vi "Periodic Tasks.vi"(8 "error in":errorcluster) -> ()   [LabVIEW 2013]
doc: "This VI runs in parallel to other tasks. It can contain as many user-defined periodic loops as you need. These can carry out PID or other sorts of timed response."
uses:
  Systems/Compressor/Compressor.lvclass
  <vilib>/Rock Robotics/SystemInterfaces/Utilities/FPGA_UtilitiesLED Source.ctl
  <vilib>/Rock Robotics/SystemInterfaces/Utilities/FPGA_UtilitiesLED State.ctl
  Systems/Blocker/Blocker.lvclass
  Commands/Command/Command.lvclass
  Systems/Catapult/Catapult.lvclass
  Systems/GrabberArms/GrabberArms.lvclass
  Systems/GrabberWheels/GrabberWheels.lvclass
  Systems/Shifter/Shifter.lvclass
  Systems/DriveMotors/DriveMotors.lvclass
  Robot Global Data.vi
panel:
  in  "Blocker Wait":u32=250
  in  "Catapult Wait":u32=75
  in  "Grabber Wait":u32=150
  in  "DriveMotors Wait":u32=75
  out "Blocker Enabled":bool
  out "Shifter Enabled":bool
  out "DML Enabled":bool
  out "DMR Enabled":bool
  out "Grabber Arms Enabled":bool
  out "Grabber Wheels Enabled":bool
  out "Catapult Enabled?":bool
  in  "System Info":T1(tab)
  out "DML":string
  out "DMR":string
  out "DML Distance":dbl
  out "DML Rate":dbl
  out "DMR Rate":dbl
  out "DMR Distance":dbl
  out "Shifter":string
  out "CT":string
  out "Catapult Switch Real Value":bool
  out "GA Switch Real Value":bool
  out "GA":string
  out "GW":string
  out "Blocker":string
  in  "Enable Catapult":bool=TRUE
  in  "Enable Grabber Wheels":bool=TRUE
  in  "Enable Grabber Arms":bool=TRUE
  in  "Enable Shifter":bool=TRUE
  in  "Enable DMR":bool=TRUE
  in  "Enable DML":bool=TRUE
  in  "Semaphore Timeout":i32=-1
  # "Manual Enables(Currently Disabled)"
  # "Dashboard Enables"
  # "Value which comes out of the DIO, which is inverted in the code"
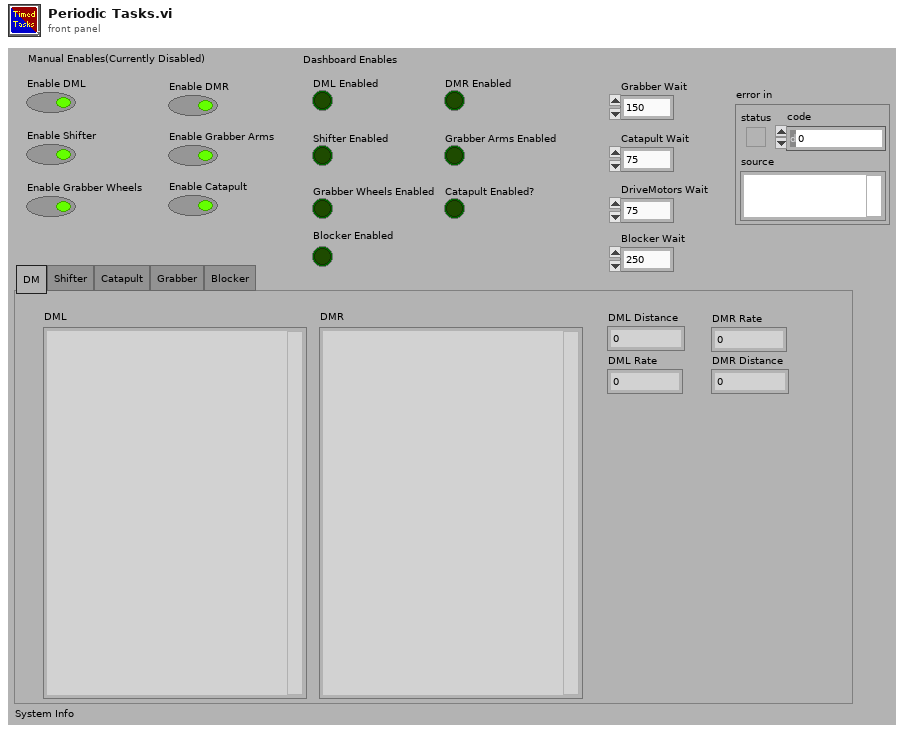
[diagram p1: front panel]
types:
  T1 = enum32{"DM", "Shifter", "Catapult", "Grabber", "Blocker"}
  T2 = typedef "Semaphore RefNum" = refnum<k1>
  T3 = typedef "WPI_DigitalInputDevRef.ctl" = cluster{"DevStatus":errorcluster, "DIO Channel":T4, "Digital Module":T5}
  T4 = typedef "FPGA_DIOChannel.ctl" = enum8{"DIO 1", "DIO 2", "DIO 3", "DIO 4", "DIO 5", "DIO 6", "DIO 7", "DIO 8", "DIO 9", "DIO 10", "DIO 11", "DIO 12", "DIO 13", "DIO 14", "Invalid"}
  T5 = typedef "FPGA_TypedefDigitalModule.ctl" = enum16{"Digital Module 1", "Digital Module 2"}
  T6 = typedef "FPGA_UtilitiesLED State.ctl" = enum16{"Off", "On", "Toggle"}
  T7 = typedef "FPGA_UtilitiesLED Source.ctl" = enum16{"User LED", "FPGA LED"}
  T8 = typedef "WPI_CompressorDevRef.ctl" = cluster{"DevStatus":errorcluster, "DigitalInputDevRef":T3, "RelayDevRef":T9}
  T9 = typedef "WPI_RelayDevRef.ctl" = cluster{"DevStatus":errorcluster, "Relay Channel":T10, "Digital Module":T5, "Relay Direction":T11}
  T10 = typedef "FPGA_DIORelayChannel.ctl" = enum8{"Relay 1", "Relay 2", "Relay 3", "Relay 4", "Relay 5", "Relay 6", "Relay 7", "Relay 8", "Invalid"}
  T11 = typedef "WPI_RelayDirection.ctl" = enum16{"Both directions", "Forward only", "Reverse only"}
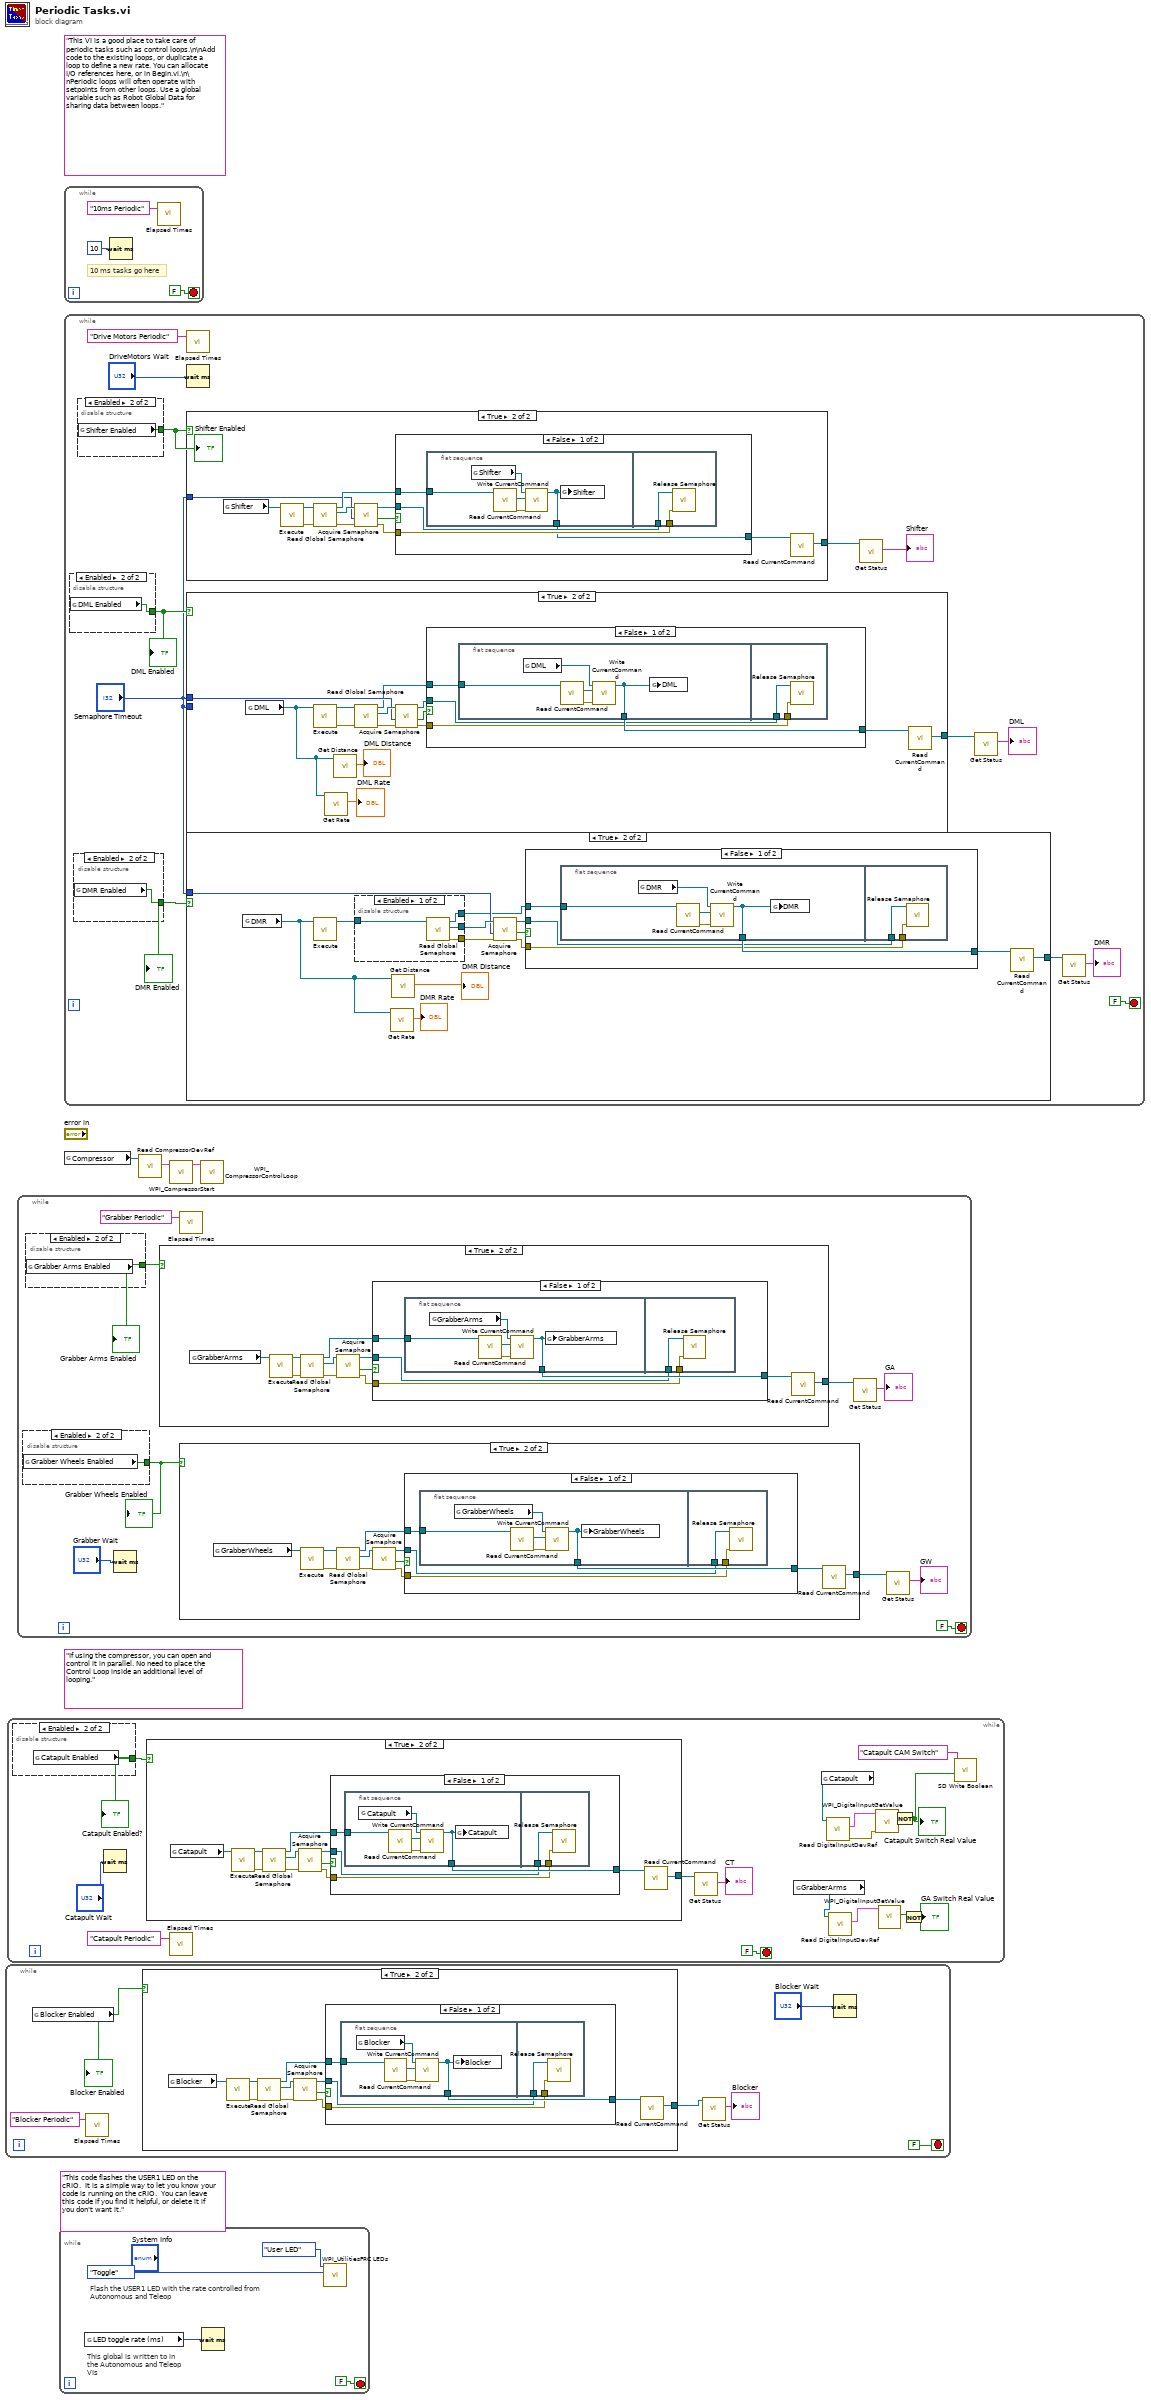
[diagram p0: block diagram]
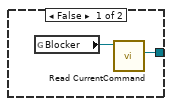
[diagram p2: hidden frame]
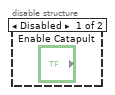
[diagram p4: hidden frame]
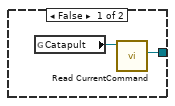
[diagram p5: hidden frame]
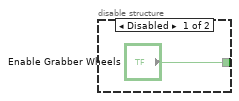
[diagram p7: hidden frame]
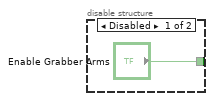
[diagram p8: hidden frame]
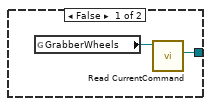
[diagram p9: hidden frame]
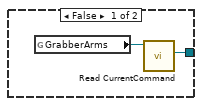
[diagram p11: hidden frame]
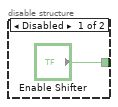
[diagram p13: hidden frame]
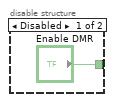
[diagram p14: hidden frame]
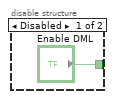
[diagram p15: hidden frame]
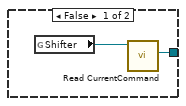
[diagram p16: hidden frame]
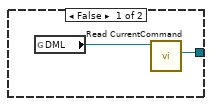
[diagram p18: hidden frame]
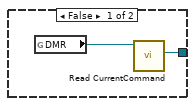
[diagram p20: hidden frame]
diagram:
  (unwired) "If using the compressor, you can open and control it in parallel. No need to place the Control Loop inside an additional level of looping."
  (unwired) "This code flashes the USER1 LED on the cRIO.  It is a simple way to let you know your code is running on the cRIO.  You can leave this code if you find it helpful, or delete it if you don't want it."
  (unwired) "This VI is a good place to take care of periodic tasks such as control loops.\n\nAdd code to the existing loops, or duplicate a loop to define a new rate. You can allocate I/O references here, or in Begin.vi.\n\nPeriodic loops will often operate with setpoints from other loops. Use a global variable such as Robot Global Data for sharing data between loops."
  n1 = while {
    stop <- FALSE stop-if-true
    n2 = global read "Robot Global Data.vi" "Blocker Enabled"() -> (w8:bool)
    "Blocker Enabled" <- w8
    n3 = call "Elapsed Times.vi"("Call Name"="Blocker Periodic") -> ()  [unwired: 2 in, 1 out]
    n4 = case shown="True" w8 {
      tunnel: [w10 w13] -> w7
      frame False {
        n5 = global read "Robot Global Data.vi" "Blocker"() -> (w11:refnum<class "Blocker.lvclass">)
        n6 = call-dynamic "Read CurrentCommand.vi"("System in"=w11) -> ("Command.lvclass"=w10:refnum<class "Command.lvclass">)  [unwired: 8 in, 2 out]
      }
      frame True {
        n7 = global read "Robot Global Data.vi" "Blocker"() -> (w22:refnum<class "Blocker.lvclass">)
        n8 = call-dynamic "Execute.vi"("System in"=w22) -> ("error out"=w20:errorcluster, "System out"=w21:refnum<class "Blocker.lvclass">)  [unwired: 9 in]
        n9 = call-dynamic "Read Global Semaphore.vi"("error in (no error)"=w20, "System in"=w21) -> ("error out"=w18:errorcluster, "semaphore"=w19:T2, "System out"=w16:refnum<class "Blocker.lvclass">)  [unwired: 7 in]
        n10 = call <vilib>:"Acquire Semaphore.vi"("error in (no error)"=w18, "semaphore"=w19) -> ("error out"=w15:errorcluster, "timed out"=w17:bool, "semaphore out"=w14:T2)  [unwired: 3 in]
        n11 = case shown="False" w17 {
          tunnel: w16 -> [w26 w34]
          tunnel: w15 -> [w23 _]
          tunnel: w14 -> [w24 _]
          tunnel: [w25 w34] -> w12
          frame False {
            n12 = flat-sequence {
              tunnel: w26 -> [w31]
              tunnel: [w27] -> w25
              tunnel: w24 -> [w33]
              tunnel: w23 -> [w32]
              frame #0 {
                n13 = global read "Robot Global Data.vi" "Blocker"() -> (w29:refnum<class "Blocker.lvclass">)
                n14 = call-dynamic "Read CurrentCommand.vi"("System in"=w31) -> ("error out"=w28:errorcluster, "Command.lvclass"=w30:refnum<class "Command.lvclass">)  [unwired: 8 in, 1 out]
                n15 = call-dynamic "Write CurrentCommand.vi"("error in (no error)"=w28, "Command.lvclass"=w30, "System in"=w29) -> ("System out"=w27:refnum<class "Blocker.lvclass">)  [unwired: 7 in, 1 out]
                n16 = global write "Robot Global Data.vi" "Blocker"(w27) -> ()
              }
              frame #1 {
                n17 = call <vilib>:"Release Semaphore.vi"("error in (no error)"=w32, "semaphore"=w33) -> ()  [unwired: 4 in, 2 out]
              }
            }
          }
          frame True {
          }
        }
        n18 = call-dynamic "Read CurrentCommand.vi"("System in"=w12) -> ("Command.lvclass"=w13:refnum<class "Command.lvclass">)  [unwired: 8 in, 2 out]
      }
    }
    n19 = call-dynamic "Get Status.vi"("Command in"=w7) -> ("Status"=→"Blocker":string)  [unwired: 8 in, 2 out]
    n20 = Wait (ms)(milliseconds to wait="Blocker Wait") -> ()  [unwired: 1 out]
  }
  n21 = while {
    stop <- FALSE stop-if-true
    n22 = disable-structure shown="Enabled" {
      disable-tunnel: [_ w51] -> w37
      frame Disabled {
      }
      frame Enabled {
        n23 = global read "Robot Global Data.vi" "Catapult Enabled"() -> (w51:bool)
      }
    }
    "Catapult Enabled?" <- w37
    n24 = Wait (ms)(milliseconds to wait="Catapult Wait") -> ()  [unwired: 1 out]
    n25 = case shown="True" w37 {
      tunnel: [w52 w55] -> w46
      frame False {
        n26 = global read "Robot Global Data.vi" "Catapult"() -> (w53:refnum<class "Catapult.lvclass">)
        n27 = call-dynamic "Read CurrentCommand.vi"("System in"=w53) -> ("Command.lvclass"=w52:refnum<class "Command.lvclass">)  [unwired: 8 in, 2 out]
      }
      frame True {
        n28 = global read "Robot Global Data.vi" "Catapult"() -> (w64:refnum<class "Catapult.lvclass">)
        n29 = call-dynamic "Execute.vi"("System in"=w64) -> ("error out"=w62:errorcluster, "System out"=w63:refnum<class "Catapult.lvclass">)  [unwired: 9 in]
        n30 = call-dynamic "Read Global Semaphore.vi"("error in (no error)"=w62, "System in"=w63) -> ("error out"=w60:errorcluster, "semaphore"=w61:T2, "System out"=w58:refnum<class "Catapult.lvclass">)  [unwired: 7 in]
        n31 = call <vilib>:"Acquire Semaphore.vi"("error in (no error)"=w60, "semaphore"=w61) -> ("error out"=w57:errorcluster, "timed out"=w59:bool, "semaphore out"=w56:T2)  [unwired: 3 in]
        n32 = case shown="False" w59 {
          tunnel: w58 -> [w68 w76]
          tunnel: w57 -> [w65 _]
          tunnel: w56 -> [w66 _]
          tunnel: [w67 w76] -> w54
          frame False {
            n33 = flat-sequence {
              tunnel: w68 -> [w73]
              tunnel: [w69] -> w67
              tunnel: w66 -> [w75]
              tunnel: w65 -> [w74]
              frame #0 {
                n34 = global read "Robot Global Data.vi" "Catapult"() -> (w71:refnum<class "Catapult.lvclass">)
                n35 = call-dynamic "Read CurrentCommand.vi"("System in"=w73) -> ("error out"=w70:errorcluster, "Command.lvclass"=w72:refnum<class "Command.lvclass">)  [unwired: 8 in, 1 out]
                n36 = call-dynamic "Write CurrentCommand.vi"("error in (no error)"=w70, "Command.lvclass"=w72, "System in"=w71) -> ("System out"=w69:refnum<class "Catapult.lvclass">)  [unwired: 7 in, 1 out]
                n37 = global write "Robot Global Data.vi" "Catapult"(w69) -> ()
              }
              frame #1 {
                n38 = call <vilib>:"Release Semaphore.vi"("error in (no error)"=w74, "semaphore"=w75) -> ()  [unwired: 4 in, 2 out]
              }
            }
          }
          frame True {
          }
        }
        n39 = call-dynamic "Read CurrentCommand.vi"("System in"=w54) -> ("Command.lvclass"=w55:refnum<class "Command.lvclass">)  [unwired: 8 in, 2 out]
      }
    }
    n40 = call "Elapsed Times.vi"("Call Name"="Catapult Periodic") -> ()  [unwired: 2 in, 1 out]
    n41 = call-dynamic "Get Status.vi"("Command in"=w46) -> ("Status"=→"CT":string)  [unwired: 8 in, 2 out]
    n42 = global read "Robot Global Data.vi" "GrabberArms"() -> (w42:refnum<class "GrabberArms.lvclass">)
    n43 = global read "Robot Global Data.vi" "Catapult"() -> (w43:refnum<class "Catapult.lvclass">)
    n44 = call-dynamic "Read DigitalInputDevRef.vi"("Catapult in"=w43) -> ("error out"=w44:errorcluster, "DigitalInputDevRef"=w45:T3)  [unwired: 8 in, 1 out]
    n45 = call-dynamic "Read DigitalInputDevRef.vi"("GrabberArms in"=w42) -> ("DigitalInputDevRef"=w41:T3)  [unwired: 8 in, 2 out]
    n46 = call <vilib>:"WPI_DigitalInputGetValue.vi"("error in (no error)"=w44, "DigitalInputDevRef"=w45) -> ("Value"=w39:bool)  [unwired: 7 in, 2 out]
    n47 = call <vilib>:"WPI_DigitalInputGetValue.vi"("DigitalInputDevRef"=w41) -> ("Value"=w40:bool)  [unwired: 8 in, 2 out]
    n48 = Not(x=w39) -> (.not. x?=w35:bool)
    "Catapult Switch Real Value" <- w35
    n49 = Not(x=w40) -> (.not. x?=→"GA Switch Real Value":bool)
    n50 = call <vilib>:"SD Write Boolean.vi"("Boolean"=w35, "Name"="Catapult CAM Switch") -> ()  [unwired: 8 in, 2 out]
  }
  n51 = while {
    stop <- FALSE stop-if-true
    n52 = disable-structure shown="Enabled" {
      disable-tunnel: ["Enable Grabber Wheels" w87] -> w77
      frame Disabled {
      }
      frame Enabled {
        n53 = global read "Robot Global Data.vi" "Grabber Wheels Enabled"() -> (w87:bool)
      }
    }
    "Grabber Wheels Enabled" <- w77
    n54 = disable-structure shown="Enabled" {
      disable-tunnel: ["Enable Grabber Arms" w89] -> w82
      frame Disabled {
      }
      frame Enabled {
        n55 = global read "Robot Global Data.vi" "Grabber Arms Enabled"() -> (w89:bool)
      }
    }
    "Grabber Arms Enabled" <- w82
    n56 = Wait (ms)(milliseconds to wait="Grabber Wait") -> ()  [unwired: 1 out]
    n57 = case shown="True" w82 {
      tunnel: [w115 w117] -> w81
      frame False {
        n58 = global read "Robot Global Data.vi" "GrabberArms"() -> (w116:refnum<class "GrabberArms.lvclass">)
        n59 = call-dynamic "Read CurrentCommand.vi"("System in"=w116) -> ("Command.lvclass"=w115:refnum<class "Command.lvclass">)  [unwired: 8 in, 2 out]
      }
      frame True {
        n60 = global read "Robot Global Data.vi" "GrabberArms"() -> (w127:refnum<class "GrabberArms.lvclass">)
        n61 = call-dynamic "Execute.vi"("System in"=w127) -> ("error out"=w125:errorcluster, "System out"=w126:refnum<class "GrabberArms.lvclass">)  [unwired: 9 in]
        n62 = call-dynamic "Read Global Semaphore.vi"("error in (no error)"=w125, "System in"=w126) -> ("error out"=w123:errorcluster, "semaphore"=w124:T2, "System out"=w121:refnum<class "GrabberArms.lvclass">)  [unwired: 7 in]
        n63 = call <vilib>:"Acquire Semaphore.vi"("error in (no error)"=w123, "semaphore"=w124) -> ("error out"=w120:errorcluster, "timed out"=w122:bool, "semaphore out"=w119:T2)  [unwired: 3 in]
        n64 = case shown="False" w122 {
          tunnel: w121 -> [w131 w139]
          tunnel: w120 -> [w128 _]
          tunnel: w119 -> [w129 _]
          tunnel: [w130 w139] -> w118
          frame False {
            n65 = flat-sequence {
              tunnel: w131 -> [w136]
              tunnel: [w132] -> w130
              tunnel: w129 -> [w138]
              tunnel: w128 -> [w137]
              frame #0 {
                n66 = global read "Robot Global Data.vi" "GrabberArms"() -> (w134:refnum<class "GrabberArms.lvclass">)
                n67 = call-dynamic "Read CurrentCommand.vi"("System in"=w136) -> ("error out"=w133:errorcluster, "Command.lvclass"=w135:refnum<class "Command.lvclass">)  [unwired: 8 in, 1 out]
                n68 = call-dynamic "Write CurrentCommand.vi"("error in (no error)"=w133, "Command.lvclass"=w135, "System in"=w134) -> ("System out"=w132:refnum<class "GrabberArms.lvclass">)  [unwired: 7 in, 1 out]
                n69 = global write "Robot Global Data.vi" "GrabberArms"(w132) -> ()
              }
              frame #1 {
                n70 = call <vilib>:"Release Semaphore.vi"("error in (no error)"=w137, "semaphore"=w138) -> ()  [unwired: 4 in, 2 out]
              }
            }
          }
          frame True {
          }
        }
        n71 = call-dynamic "Read CurrentCommand.vi"("System in"=w118) -> ("Command.lvclass"=w117:refnum<class "Command.lvclass">)  [unwired: 8 in, 2 out]
      }
    }
    n72 = call "Elapsed Times.vi"("Call Name"="Grabber Periodic") -> ()  [unwired: 2 in, 1 out]
    n73 = case shown="True" w77 {
      tunnel: [w90 w92] -> w79
      frame False {
        n74 = global read "Robot Global Data.vi" "GrabberWheels"() -> (w91:refnum<class "GrabberWheels.lvclass">)
        n75 = call-dynamic "Read CurrentCommand.vi"("System in"=w91) -> ("Command.lvclass"=w90:refnum<class "Command.lvclass">)  [unwired: 8 in, 2 out]
      }
      frame True {
        n76 = global read "Robot Global Data.vi" "GrabberWheels"() -> (w102:refnum<class "GrabberWheels.lvclass">)
        n77 = call-dynamic "Execute.vi"("System in"=w102) -> ("error out"=w100:errorcluster, "System out"=w101:refnum<class "GrabberWheels.lvclass">)  [unwired: 9 in]
        n78 = call-dynamic "Read Global Semaphore.vi"("error in (no error)"=w100, "System in"=w101) -> ("error out"=w98:errorcluster, "semaphore"=w99:T2, "System out"=w96:refnum<class "GrabberWheels.lvclass">)  [unwired: 7 in]
        n79 = call <vilib>:"Acquire Semaphore.vi"("error in (no error)"=w98, "semaphore"=w99) -> ("error out"=w95:errorcluster, "timed out"=w97:bool, "semaphore out"=w94:T2)  [unwired: 3 in]
        n80 = case shown="False" w97 {
          tunnel: w96 -> [w106 w114]
          tunnel: w95 -> [w103 _]
          tunnel: w94 -> [w104 _]
          tunnel: [w105 w114] -> w93
          frame False {
            n81 = flat-sequence {
              tunnel: w106 -> [w111]
              tunnel: [w107] -> w105
              tunnel: w104 -> [w113]
              tunnel: w103 -> [w112]
              frame #0 {
                n82 = global read "Robot Global Data.vi" "GrabberWheels"() -> (w109:refnum<class "GrabberWheels.lvclass">)
                n83 = call-dynamic "Read CurrentCommand.vi"("System in"=w111) -> ("error out"=w108:errorcluster, "Command.lvclass"=w110:refnum<class "Command.lvclass">)  [unwired: 8 in, 1 out]
                n84 = call-dynamic "Write CurrentCommand.vi"("error in (no error)"=w108, "Command.lvclass"=w110, "System in"=w109) -> ("System out"=w107:refnum<class "GrabberWheels.lvclass">)  [unwired: 7 in, 1 out]
                n85 = global write "Robot Global Data.vi" "GrabberWheels"(w107) -> ()
              }
              frame #1 {
                n86 = call <vilib>:"Release Semaphore.vi"("error in (no error)"=w112, "semaphore"=w113) -> ()  [unwired: 4 in, 2 out]
              }
            }
          }
          frame True {
          }
        }
        n87 = call-dynamic "Read CurrentCommand.vi"("System in"=w93) -> ("Command.lvclass"=w92:refnum<class "Command.lvclass">)  [unwired: 8 in, 2 out]
      }
    }
    n88 = call-dynamic "Get Status.vi"("Command in"=w81) -> ("Status"=→"GA":string)  [unwired: 8 in, 2 out]
    n89 = call-dynamic "Get Status.vi"("Command in"=w79) -> ("Status"=→"GW":string)  [unwired: 8 in, 2 out]
  }
  n90 = while {
    stop <- FALSE stop-if-true
    # "This global is written to in the Autonomous and Teleop VIs"
    # "Flash the USER1 LED with the rate controlled from Autonomous and Teleop"
    n91 = global read "Robot Global Data.vi" "LED toggle rate (ms)"() -> (w140:u32)
    n92 = Wait (ms)(milliseconds to wait=w140) -> ()  [unwired: 1 out]
    n93 = call <vilib>:"WPI_UtilitiesFRC LEDs.vi"("State"=FPGA_UtilitiesLED_State."Toggle", "LED Type"=FPGA_UtilitiesLED_Source."User LED") -> ()  [unwired: 1 in, 9 out]
  }
  n94 = while {
    stop <- FALSE stop-if-true
    # "10 ms tasks go here"
    n95 = Wait (ms)(milliseconds to wait=u32 10) -> ()  [unwired: 1 out]
    n96 = call "Elapsed Times.vi"("Call Name"="10ms Periodic") -> ()  [unwired: 2 in, 1 out]
  }
  n97 = while {
    stop <- FALSE stop-if-true
    n98 = disable-structure shown="Enabled" {
      disable-tunnel: ["Enable DMR" w163] -> w151
      frame Disabled {
      }
      frame Enabled {
        n99 = global read "Robot Global Data.vi" "DML Enabled"() -> (w163:bool)
      }
    }
    "DML Enabled" <- w151
    n100 = disable-structure shown="Enabled" {
      disable-tunnel: ["Enable DML" w165] -> w154
      frame Disabled {
      }
      frame Enabled {
        n101 = global read "Robot Global Data.vi" "DMR Enabled"() -> (w165:bool)
      }
    }
    "DMR Enabled" <- w154
    n102 = disable-structure shown="Enabled" {
      disable-tunnel: ["Enable Shifter" w161] -> w148
      frame Disabled {
      }
      frame Enabled {
        n103 = global read "Robot Global Data.vi" "Shifter Enabled"() -> (w161:bool)
      }
    }
    "Shifter Enabled" <- w148
    n104 = call "Elapsed Times.vi"("Call Name"="Drive Motors Periodic") -> ()  [unwired: 2 in, 1 out]
    n105 = Wait (ms)(milliseconds to wait="DriveMotors Wait") -> ()  [unwired: 1 out]
    n106 = case shown="True" w148 {
      tunnel: [w167 w175] -> w150
      tunnel: "Semaphore Timeout" -> [_ w169]
      frame False {
        n107 = global read "Robot Global Data.vi" "Shifter"() -> (w166:refnum<class "Shifter.lvclass">)
        n108 = call-dynamic "Read CurrentCommand.vi"("System in"=w166) -> ("Command.lvclass"=w167:refnum<class "Command.lvclass">)  [unwired: 8 in, 2 out]
      }
      frame True {
        n109 = global read "Robot Global Data.vi" "Shifter"() -> (w170:refnum<class "Shifter.lvclass">)
        n110 = call-dynamic "Execute.vi"("System in"=w170) -> ("error out"=w171:errorcluster, "System out"=w172:refnum<class "Shifter.lvclass">)  [unwired: 9 in]
        n111 = call-dynamic "Read Global Semaphore.vi"("error in (no error)"=w171, "System in"=w172) -> ("error out"=w168:errorcluster, "semaphore"=w179:T2, "System out"=w178:refnum<class "Shifter.lvclass">)  [unwired: 7 in]
        n112 = call <vilib>:"Acquire Semaphore.vi"("error in (no error)"=w168, "ms timeout (-1)"=w169, "semaphore"=w179) -> ("error out"=w173:errorcluster, "timed out"=w177:bool, "semaphore out"=w174:T2)  [unwired: 2 in]
        n113 = case shown="False" w177 {
          tunnel: w178 -> [w181 w191]
          tunnel: [w180 w191] -> w176
          tunnel: w174 -> [w183 _]
          tunnel: w173 -> [w182 _]
          frame False {
            n114 = flat-sequence {
              tunnel: w181 -> [w186]
              tunnel: [w185] -> w180
              tunnel: w183 -> [w190]
              tunnel: w182 -> [w189]
              frame #0 {
                n115 = global read "Robot Global Data.vi" "Shifter"() -> (w187:refnum<class "Shifter.lvclass">)
                n116 = call-dynamic "Read CurrentCommand.vi"("System in"=w186) -> ("error out"=w188:errorcluster, "Command.lvclass"=w184:refnum<class "Command.lvclass">)  [unwired: 8 in, 1 out]
                n117 = call-dynamic "Write CurrentCommand.vi"("error in (no error)"=w188, "Command.lvclass"=w184, "System in"=w187) -> ("System out"=w185:refnum<class "Shifter.lvclass">)  [unwired: 7 in, 1 out]
                n118 = global write "Robot Global Data.vi" "Shifter"(w185) -> ()
              }
              frame #1 {
                n119 = call <vilib>:"Release Semaphore.vi"("error in (no error)"=w189, "semaphore"=w190) -> ()  [unwired: 4 in, 2 out]
              }
            }
          }
          frame True {
          }
        }
        n120 = call-dynamic "Read CurrentCommand.vi"("System in"=w176) -> ("Command.lvclass"=w175:refnum<class "Command.lvclass">)  [unwired: 8 in, 2 out]
      }
    }
    n121 = case shown="True" w151 {
      tunnel: "Semaphore Timeout" -> [_ _]
      tunnel: [w193 w201] -> w152
      tunnel: "Semaphore Timeout" -> [_ w205]
      frame False {
        n122 = global read "Robot Global Data.vi" "DML"() -> (w192:refnum<class "DriveMotors.lvclass">)
        n123 = call-dynamic "Read CurrentCommand.vi"("System in"=w192) -> ("Command.lvclass"=w193:refnum<class "Command.lvclass">)  [unwired: 8 in, 2 out]
      }
      frame True {
        n124 = global read "Robot Global Data.vi" "DML"() -> (w194:refnum<class "DriveMotors.lvclass">)
        n125 = call-dynamic "Execute.vi"("System in"=w194) -> ("error out"=w199:errorcluster, "System out"=w207:refnum<class "DriveMotors.lvclass">)  [unwired: 9 in]
        n126 = call-dynamic "Get Rate.vi"("DriveMotors in"=w194) -> ("Rate"=→"DML Rate":dbl)  [unwired: 8 in, 2 out]
        n127 = call-dynamic "Get Distance.vi"("DriveMotors in"=w194) -> ("Distance"=→"DML Distance":dbl)  [unwired: 8 in, 2 out]
        n128 = call-dynamic "Read Global Semaphore.vi"("error in (no error)"=w199, "System in"=w207) -> ("error out"=w198:errorcluster, "semaphore"=w206:T2, "System out"=w203:refnum<class "DriveMotors.lvclass">)  [unwired: 7 in]
        n129 = call <vilib>:"Acquire Semaphore.vi"("error in (no error)"=w198, "ms timeout (-1)"=w205, "semaphore"=w206) -> ("error out"=w197:errorcluster, "timed out"=w204:bool, "semaphore out"=w200:T2)  [unwired: 2 in]
        n130 = case shown="False" w204 {
          tunnel: w203 -> [w211 w219]
          tunnel: [w210 w219] -> w202
          tunnel: w200 -> [w208 _]
          tunnel: w197 -> [w209 _]
          frame False {
            n131 = flat-sequence {
              tunnel: w211 -> [w213]
              tunnel: [w212] -> w210
              tunnel: w209 -> [w218]
              tunnel: w208 -> [w217]
              frame #0 {
                n132 = global read "Robot Global Data.vi" "DML"() -> (w216:refnum<class "DriveMotors.lvclass">)
                n133 = call-dynamic "Read CurrentCommand.vi"("System in"=w213) -> ("error out"=w215:errorcluster, "Command.lvclass"=w214:refnum<class "Command.lvclass">)  [unwired: 8 in, 1 out]
                n134 = call-dynamic "Write CurrentCommand.vi"("error in (no error)"=w215, "Command.lvclass"=w214, "System in"=w216) -> ("System out"=w212:refnum<class "DriveMotors.lvclass">)  [unwired: 7 in, 1 out]
                n135 = global write "Robot Global Data.vi" "DML"(w212) -> ()
              }
              frame #1 {
                n136 = call <vilib>:"Release Semaphore.vi"("error in (no error)"=w218, "semaphore"=w217) -> ()  [unwired: 4 in, 2 out]
              }
            }
          }
          frame True {
          }
        }
        n137 = call-dynamic "Read CurrentCommand.vi"("System in"=w202) -> ("Command.lvclass"=w201:refnum<class "Command.lvclass">)  [unwired: 8 in, 2 out]
      }
    }
    n138 = case shown="True" w154 {
      tunnel: "Semaphore Timeout" -> [_ w227]
      tunnel: [w221 w228] -> w155
      frame False {
        n139 = global read "Robot Global Data.vi" "DMR"() -> (w220:refnum<class "DriveMotors.lvclass">)
        n140 = call-dynamic "Read CurrentCommand.vi"("System in"=w220) -> ("Command.lvclass"=w221:refnum<class "Command.lvclass">)  [unwired: 8 in, 2 out]
      }
      frame True {
        n141 = global read "Robot Global Data.vi" "DMR"() -> (w222:refnum<class "DriveMotors.lvclass">)
        n142 = call-dynamic "Execute.vi"("System in"=w222) -> ("System out"=w226:refnum<class "DriveMotors.lvclass">)  [unwired: 9 in, 1 out]
        n143 = disable-structure shown="Enabled" {
          disable-tunnel: [w238 w241] -> w234
          disable-tunnel: [w237 w240] -> w233
          disable-tunnel: w226 -> [w236 w242]
          disable-tunnel: [w235 w242] -> w225
          frame Enabled {
            n144 = call-dynamic "Read Global Semaphore.vi"("System in"=w236) -> ("error out"=w237:errorcluster, "semaphore"=w238:T2, "System out"=w235:refnum<class "DriveMotors.lvclass">)  [unwired: 8 in]
          }
          frame Disabled {
            n145 = call <vilib>:"Get LV Class Name.vi"("object"=w242) -> ("class name"=w239:string)  [unwired: 9 in, 1 out]
            n146 = call <vilib>:"Obtain Semaphore Reference.vi"("name (unnamed)"=w239) -> ("error out"=w240:errorcluster, "semaphore"=w241:T2)  [unwired: 4 in, 1 out]
          }
        }
        n147 = call-dynamic "Get Rate.vi"("DriveMotors in"=w222) -> ("Rate"=→"DMR Rate":dbl)  [unwired: 8 in, 2 out]
        n148 = call-dynamic "Get Distance.vi"("DriveMotors in"=w222) -> ("Distance"=→"DMR Distance":dbl)  [unwired: 8 in, 2 out]
        n149 = call <vilib>:"Acquire Semaphore.vi"("error in (no error)"=w233, "ms timeout (-1)"=w227, "semaphore"=w234) -> ("error out"=w230:errorcluster, "timed out"=w232:bool, "semaphore out"=w231:T2)  [unwired: 2 in]
        n150 = case shown="False" w232 {
          tunnel: w225 -> [w246 w254]
          tunnel: w231 -> [w244 _]
          tunnel: w230 -> [w243 _]
          tunnel: [w245 w254] -> w229
          frame False {
            n151 = flat-sequence {
              tunnel: w246 -> [w250]
              tunnel: [w247] -> w245
              tunnel: w244 -> [w253]
              tunnel: w243 -> [w252]
              frame #0 {
                n152 = global read "Robot Global Data.vi" "DMR"() -> (w251:refnum<class "DriveMotors.lvclass">)
                n153 = call-dynamic "Read CurrentCommand.vi"("System in"=w250) -> ("error out"=w249:errorcluster, "Command.lvclass"=w248:refnum<class "Command.lvclass">)  [unwired: 8 in, 1 out]
                n154 = call-dynamic "Write CurrentCommand.vi"("error in (no error)"=w249, "Command.lvclass"=w248, "System in"=w251) -> ("System out"=w247:refnum<class "DriveMotors.lvclass">)  [unwired: 7 in, 1 out]
                n155 = global write "Robot Global Data.vi" "DMR"(w247) -> ()
              }
              frame #1 {
                n156 = call <vilib>:"Release Semaphore.vi"("error in (no error)"=w252, "semaphore"=w253) -> ()  [unwired: 4 in, 2 out]
              }
            }
          }
          frame True {
          }
        }
        n157 = call-dynamic "Read CurrentCommand.vi"("System in"=w229) -> ("Command.lvclass"=w228:refnum<class "Command.lvclass">)  [unwired: 8 in, 2 out]
      }
    }
    n158 = call-dynamic "Get Status.vi"("Command in"=w150) -> ("Status"=→"Shifter":string)  [unwired: 8 in, 2 out]
    n159 = call-dynamic "Get Status.vi"("Command in"=w152) -> ("Status"=→"DML":string)  [unwired: 8 in, 2 out]
    n160 = call-dynamic "Get Status.vi"("Command in"=w155) -> ("Status"=→"DMR":string)  [unwired: 8 in, 2 out]
  }
  n161 = global read "Robot Global Data.vi" "Compressor"() -> (w3:refnum<class "Compressor.lvclass">)
  n162 = call-dynamic "Read CompressorDevRef.vi"("Compressor in"=w3) -> ("CompressorDevRef"=w2:T8)  [unwired: 8 in, 2 out]
  n163 = call <vilib>:"WPI_CompressorStart.vi"("CompressorDevRef"=w2) -> ("CompressorDevRef"=w1:T8)  [unwired: 9 in, 1 out]
  n164 = call <vilib>:"WPI_CompressorControlLoop.vi"("CompressorDevRef"=w1) -> ()  [unwired: 11 in]
